vi "Joystick Button States.vi"(11 "buttons":bool[](array[boolean])) -> (0 "just released":bool[](array[boolean]), 1 "just pressed":bool[](array[boolean]), 2 "down":bool[](array[boolean]), 3 "up":bool[](array[boolean]))   [LabVIEW 2026]
doc: "This VI compares the button values to previous and identifies four common states."
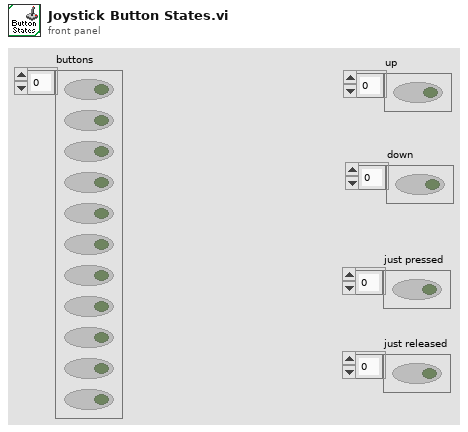
[diagram p1: front panel]
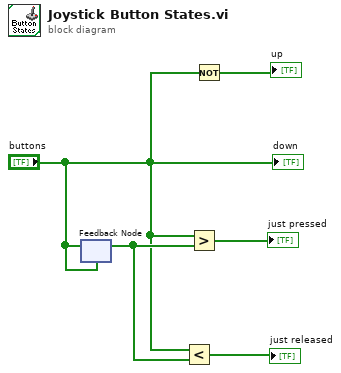
[diagram p0: block diagram]
diagram:
  n1 = feedback-in #1("buttons") -> ()
  n2 = feedback #1("buttons") -> (w3:bool[])
  n3 = Less?(x="buttons", y=w3) -> (x < y?=→"just released":bool[])
  n4 = Greater?(x="buttons", y=w3) -> (0:→"just pressed":bool[])
  n5 = Not(x="buttons") -> (.not. x?=→"up":bool[])
  "down" <- "buttons"
